vi "Test_Benchmarking_LocalLogEventCallNotInitialized_AvgCallTimeSub10uS.vi"(8 "error in (no error)":errorcluster, 11 "Benchmarking in":refnum<class "Benchmarking.lvclass">) -> (0 "error out":errorcluster, 3 "Benchmarking out":refnum<class "Benchmarking.lvclass">)   [LabVIEW 2017, in "Benchmarking.lvclass"]
uses:
  Benchmarking.lvclass
  Source/Composed Log/LoggerReference/LoggerReference.lvclass/LoggerReference.ctl
  Source/Composed Log/Types/Log Level.ctl
  c732dfe6-6ae6-40e1-b7d0-4452a78b430e.vi
  <vilib>/Analysis/baseanly.llb/Mean (DBL).vi
  Source/Composed Log/LoggerReference/Return Aggregate Queues.vi
  Source/Composed Log/LoggerReference/Add Aggregate Log.vi
  c732dfe6-6ae6-40e1-b7d0-4452a78b430e.vi/b90949e6-ac07-4381-bf2f-417c398e7aa0.vi
  Source/Composed Log/LoggerReference/Log.vi
  Source/Composed Log/LoggerReference/Get Valid Event Time.vi
  Source/Composed Log/LoggerReference/Send Add Sink.vi
  Source/Composed Log/LoggerReference/Remove Stale Logs.vi
  Source/Composed Log/Application Logger/Launch Worker Loop.vi
  Source/Composed Log/LoggerReference/Initialize Logger Instance.vi
  Source/Composed Log/Log Sink/Log Sink.lvclass
  Source/Composed Log/LoggerReference/LoggerReference.lvclass
  Source/Composed Log/IErrorFormat/IErrorFormat.lvclass
  Source/Composed Log/Composed Log.lvlib
  <vilib>/Analysis/NI_AALBase.lvlib
  <vilib>/addons/_JKI Toolkits/VI Tester/TestCase.llb/TestCase.lvclass
  C:/Program Files (x86)/National Instruments/LabVIEW 2017/vi.lib/addons/_JKI Toolkits/VI Tester/TestCase.llb/TestCase.lvclass
panel:
  in  "Numeric":i32=10000
  out "min index(es)":i32
  out "max index(es)":i32
  out "Histogram Graph":T1(graph)
  out "Benchmark Results":string
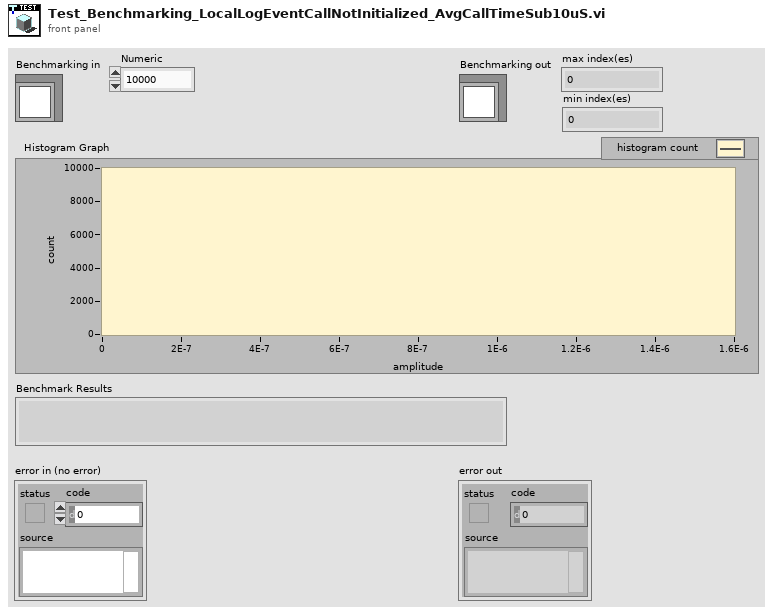
[diagram p1: front panel]
types:
  T1 = cluster{"X Values":dbl[], "Histogram: h(x)":i32[]}
  T2 = typedef "Composed Log.lvlib/Log Level.ctl" = enum16{"Debug", "Info", "Warning", "Error", "Critical"}
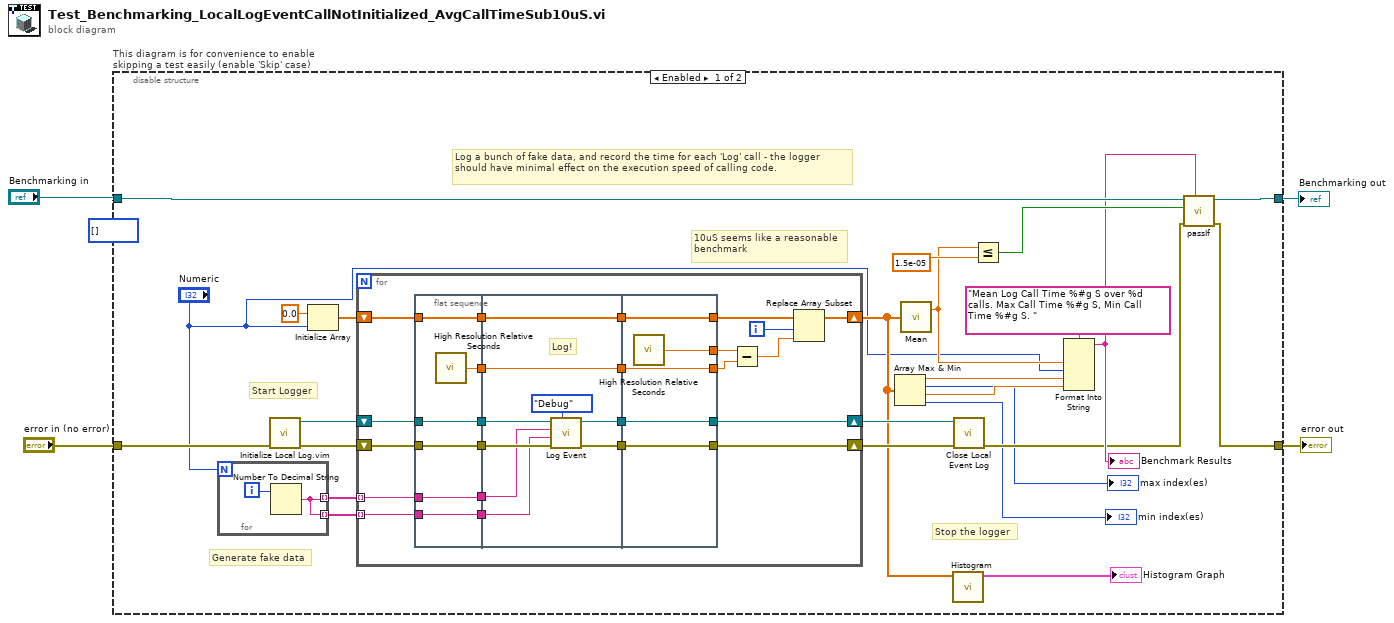
[diagram p0: block diagram]
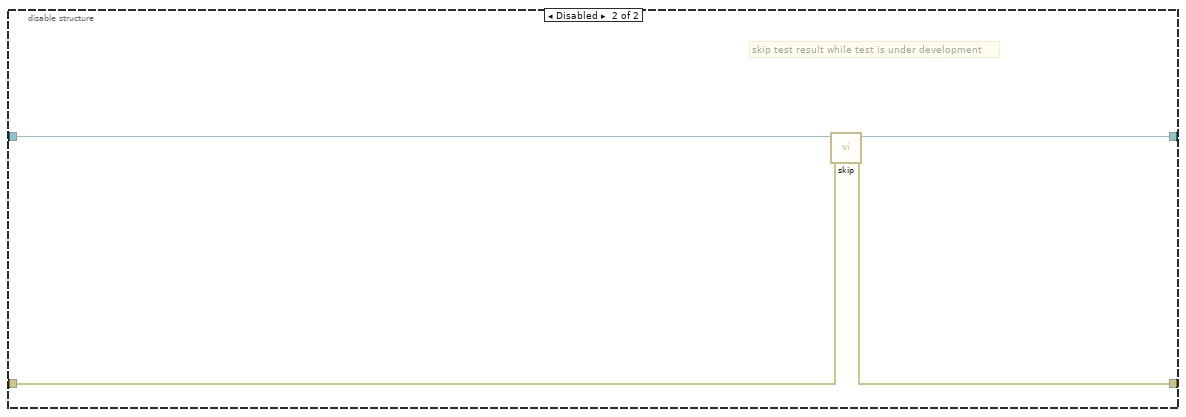
[diagram p2: hidden frame]
diagram:
  n1 = disable-structure "This diagram is for convenience to enable skipping a test easily (enable 'Skip' case)" shown="Enabled" {
    disable-tunnel: "Benchmarking in" -> [w28 w78]
    disable-tunnel: [w27 w76] -> w4
    disable-tunnel: [w29 w77] -> w3
    disable-tunnel: "error in (no error)" -> [w26 w75]
    frame Enabled {
      (unwired) i32[] []
      # "Stop the logger"
      # "10uS seems like a reasonable    benchmark"
      # "Generate fake data"
      # "Start Logger"
      # "Log a bunch of fake data, and record the time for each 'Log' call - the logger should have minimal effect on the execution speed of calling code."
      n2 = for {
        N: "Numeric" -> [_]
        tunnel: [w73] -> w25 mode=indexing
        tunnel: [w73] -> w22 mode=indexing
        i -> [w74]
        n3 = Number To Decimal String(number=w74) -> (decimal integer string=w73:string)  [unwired: 1 in]
      }
      n4 = call "Initialize Local Log.vim"("error in (no error)"=w26) -> ("error out"=w13:errorcluster, "Log Instance Reference"=w12:refnum<class "LoggerReference.lvclass">)  [unwired: 8 in, 1 out]
      n5 = Initialize Array(0.0 ("element"), "Numeric") -> (w23:dbl[])
      n6 = for {
        tunnel: w25 -> [w47] mode=indexing
        shift-right: [w45] -> w15
        shift-left: w13 -> [w46]
        shift-right: [w36] -> w10
        shift-left: w23 -> [w42]
        tunnel: w22 -> [w35] mode=indexing
        shift-right: [w31] -> w11
        shift-left: w12 -> [w30]
        i -> [w38]
        n7 = flat-sequence {
          tunnel: w46 -> [w57]
          tunnel: w47 -> [w58]
          tunnel: [w58] -> w52
          tunnel: [w57] -> w51
          tunnel: [w56] -> w50
          tunnel: w42 -> [w55]
          tunnel: [w55] -> w40
          tunnel: w35 -> [w54]
          tunnel: [w54] -> w34
          tunnel: [w53] -> w33
          tunnel: w30 -> [w53]
          tunnel: w52 -> [w63]
          tunnel: w51 -> [w67]
          tunnel: w50 -> [w65]
          tunnel: [w66] -> w49
          tunnel: [w65] -> w48
          tunnel: [w64] -> w41
          tunnel: w40 -> [w64]
          tunnel: w34 -> [w62]
          tunnel: w33 -> [w61]
          tunnel: [w60] -> w32
          tunnel: [w71] -> w44
          tunnel: [w72] -> w45
          tunnel: w49 -> [w72]
          tunnel: w48 -> [w71]
          tunnel: [w70] -> w43
          tunnel: [w69] -> w39
          tunnel: w41 -> [w69]
          tunnel: w32 -> [w68]
          tunnel: [w68] -> w31
          frame #0 {
            n8 = call <vilib>:"High Resolution Relative Seconds.vi"() -> ("relative seconds"=w56:dbl)
          }
          frame #1 {
            # "Log!"
            n9 = call "Log Event.vi"("Event Level"=Log_Level."Debug", "error in (no error)"=w67, "Data To Log"=w62, "SourceID"=w63, "Log Instance"=w61) -> ("error out"=w66:errorcluster, "Log Instance Out"=w60:refnum<class "LoggerReference.lvclass">)  [unwired: 5 in]
          }
          frame #2 {
            n10 = call <vilib>:"High Resolution Relative Seconds.vi"() -> ("relative seconds"=w70:dbl)
          }
        }
        n11 = Subtract(x=w43, y=w44) -> (x-y=w37:dbl)
        n12 = Replace Array Subset(array=w39, new element=w37, index=w38) -> (w36:dbl[])
      }
      n13 = Array Max & Min(array=w10) -> (max value=w18:dbl, max index (indices)=→"max index(es)":i32, min value=w17:dbl, min index (indices)=→"min index(es)":i32)
      n14 = call-poly <vilib>:"Mean.vi"("X"=w10) -> ("mean"=w7:dbl)  [unwired: 1 out]
      n15 = call <vilib>:"Histogram.vi"("X"=w10) -> ("Histogram Graph"=→"Histogram Graph":T1)  [unwired: 7 in, 3 out]
      n16 = call "Close Local Event Log.vi"("error in (no error)"=w15, "Log Instance"=w11) -> ("error out"=w14:errorcluster)  [unwired: 9 in]
      n17 = Less Or Equal?(x=w7, y=1.5e-05) -> (x <= y?=w20:bool)
      n18 = Format Into String(format string="Mean Log Call Time %#g S over %d calls. Max Call Time %#g S, Min Call Time %#g S. ", w7, "Numeric", w18, w17) -> (resulting string=w16:string)  [unwired: 2 in, 1 out]
      "Benchmark Results" <- w16
      n19 = call-dynamic "passIf.vi"("custom report message (\"\")"=w16, "error in (no error)"=w14, "pass"=w20, "TestCase in"=w28) -> ("error out"=w29:errorcluster, "TestCase out"=w27:refnum<class "Benchmarking.lvclass">)  [unwired: 6 in]
    }
    frame Disabled {
      # "skip test result while test is under development"
      n20 = call <vilib>:"skip.vi"("error in (no error)"=w75, "TestCase in"=w78) -> ("error out"=w77:errorcluster, "TestCase out"=w76:refnum<class "Benchmarking.lvclass">)  [unwired: 8 in]
    }
  }
  "error out" <- w3
  "Benchmarking out" <- w4
